vi "database_connection_write.vi"(5 "ODBC data source name":string="amrc_monitoring", 6 "error in (no error)":errorcluster, 7 "G1?":u32, 8 "current time":timestamp, 9 "data 2":dbl[](array[numeric]), 10 "Machine Data":T1={"Zload"="", "Yload"="", "Xload"="", "path_position"="", "Fovr"="", "SspeedOvr"="", "Program Name"="", "Program status"="", "Block of code being executed"="", "Line of code"="", "Machine availability"="", "Emergency status"="", "Controller mode"="", "Tool_id"="UNAVAILABLE"}, 11 "Machine type":string) -> (3 "error out":errorcluster)   [LabVIEW 2017]
uses:
  <vilib>/addons/database/Connection.llb/DB Tools Open Connec (String).vi
  <vilib>/addons/database/Connection.llb/Conn Execute.vi
  <vilib>/addons/database/Recordset.llb/Rec Destroy - Connection.vi
  <vilib>/addons/database/NI_Database_API.lvlib
panel:
  out "Tool_id":string
  out "resulting string":string
  out "size(s)":i32
  out "concatenated string 5":string
  out "concatenated string 4":string
  out "concatenated string 3":string
  out "concatenated string 2":string
  out "concatenated string":string
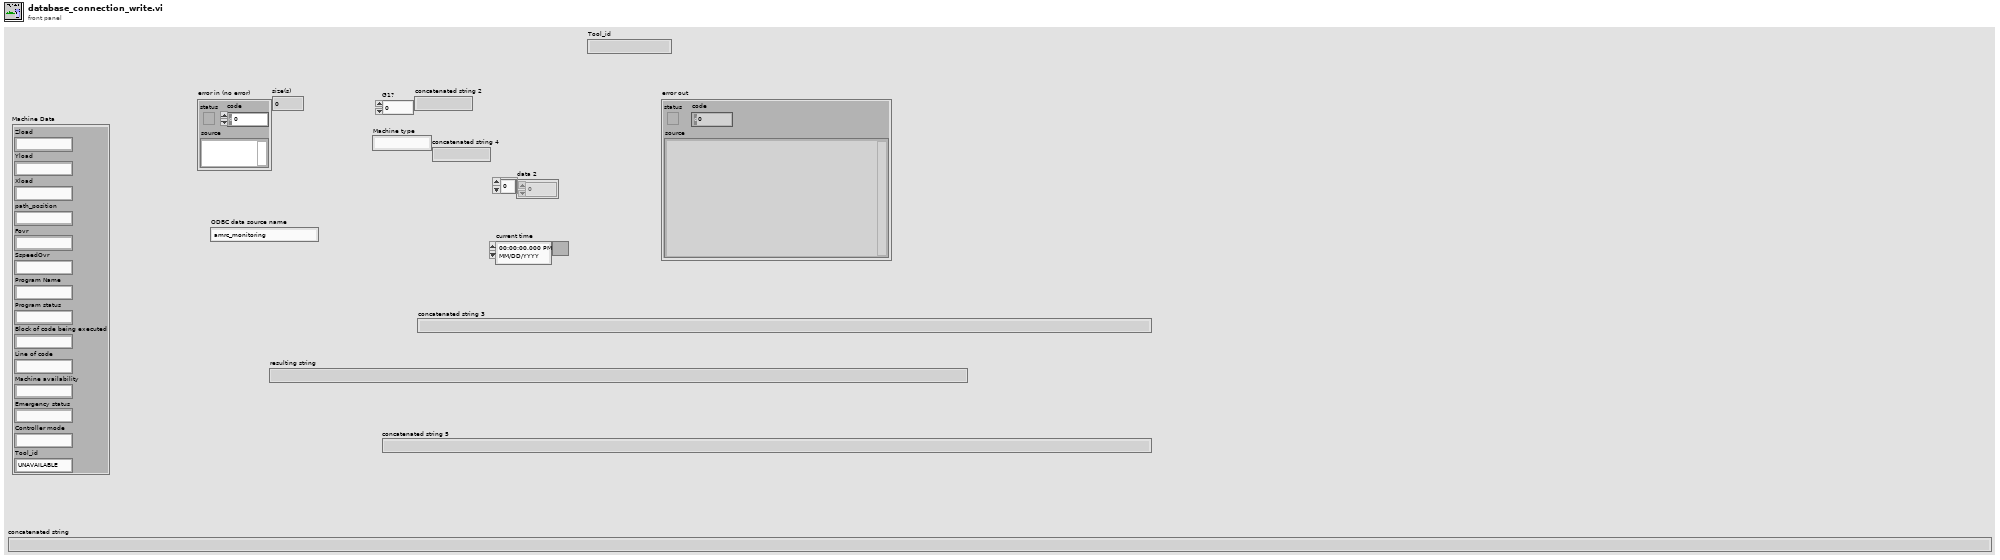
[diagram p1: front panel]
types:
  T1 = cluster{"Zload":string, "Yload":string, "Xload":string, "path_position":string, "Fovr":string, "SspeedOvr":string, "Program Name":string, "Program status":string, "Block of code being executed":string, "Line of code":string, "Machine availability":string, "Emergency status":string, "Controller mode":string, "Tool_id":string}
  T2 = typedef "NI_Database_API.lvlib/Conn ObjectReference.ctl" = refnum<k1>
  T3 = typedef "NI_Database_API.lvlib/Rec ObjectReference.ctl" = refnum<k1>
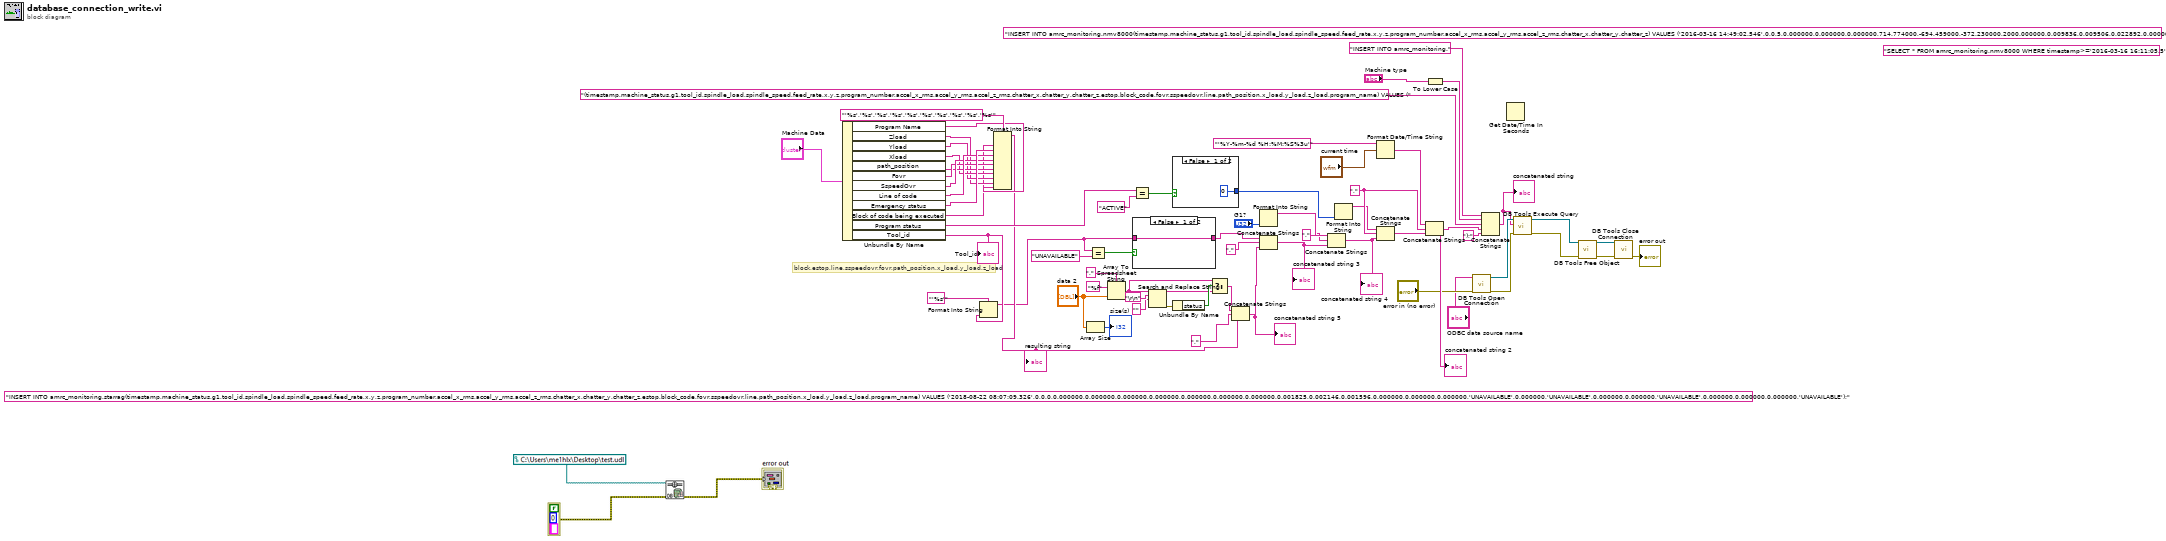
[diagram p0: block diagram]
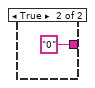
[diagram p2: hidden frame]
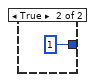
[diagram p3: hidden frame]
diagram:
  (unwired) "INSERT INTO amrc_monitoring.starrag(timestamp,machine_status,g1,tool_id,spindle_load,spindle_speed,feed_rate,x,y,z,program_number,accel_x_rms,accel_y_rms,accel_z_rms,chatter_x,chatter_y,chatter_z,estop,block_code,fovr,sspeedovr,line,path_position,x_load,y_load,z_load,program_name) VALUES ('2018-08-22 08:07:09.326',0,0,0,0.000000,0.000000,0.000000,0.000000,0.000000,0.000000,0.000000,0.001825,0.002146,0.001596,0.000000,0.000000,0.000000,'UNAVAILABLE',0.000000,'UNAVAILABLE',0.000000,0.000000,'UNAVAILABLE',0.000000,0.000000,0.000000,'UNAVAILABLE');" ("string")
  w47 = "," ("string")
  (unwired) "SELECT * FROM amrc_monitoring.nmv8000 WHERE timestamp>='2016-03-16 16:11:05.5' " ("SQL query")
  (unwired) "INSERT INTO amrc_monitoring.nmv8000(timestamp,machine_status,g1,tool_id,spindle_load,spindle_speed,feed_rate,x,y,z,program_number,accel_x_rms,accel_y_rms,accel_z_rms,chatter_x,chatter_y,chatter_z) VALUES ('2016-03-16 14:49:02.546',0,0,5,0.000000,0.000000,0.000000,714.774000,-694.459000,-372.230000,2000.000000,0.009836,0.009506,0.022892,0.000000,1.000000,0.000000);" ("SQL query")
  # "block,estop,line,sspeedovr,fovr,path_position,x_load,y_load,z_load"
  n1 = Unbundle By Name("Machine Data") -> ("Program Name"=w16:string, "Zload"=w21:string, "Yload"=w22:string, "Xload"=w23:string, "path_position"=w24:string, "Fovr"=w25:string, "SspeedOvr"=w26:string, "Line of code"=w27:string, "Emergency status"=w28:string, "Block of code being executed"=w12:string, "Program status"=w57:string, "Tool_id"=w2:string)
  "Tool_id" <- w2
  n2 = Format Into String(format string="'%s'", w2) -> (resulting string=w1:string)  [unwired: 2 in, 1 out]
  n3 = Format Into String(format string="'%s','%s','%s','%s','%s','%s','%s','%s','%s','%s'", w12, w28, w27, w26, w25, w24, w23, w22, w21, w16) -> (resulting string=w6:string)  [unwired: 2 in, 1 out]
  "resulting string" <- w6
  n4 = Array Size(array="data 2") -> (size(s)=→"size(s)":i32)
  n5 = Equal?(x=w1, y="UNAVAILABLE") -> (x = y?=w53:bool)
  n6 = Array To Spreadsheet String(delimiter (Tab)=",", array="data 2", 3:"%f" ("format string")) -> (spreadsheet string=w38:string)
  n7 = case shown="False" w53 {
    tunnel: w1 -> [w65 _]
    tunnel: [w65 "0"] -> w4
    frame False {
    }
    frame True {
    }
  }
  n8 = Equal?(x=w57, y="ACTIVE") -> (x = y?=w55:bool)
  n9 = Search and Replace String(input string=w38, search string="\r\n", replace string="" ("replace string (\"\")")) -> (result string=w39:string, error out=w41:errorcluster)  [unwired: 5 in, 2 out]
  n10 = case shown="False" w55 {
    tunnel: [0 1] -> w54
    frame False {
    }
    frame True {
    }
  }
  n11 = Unbundle By Name(w41) -> ("status"=w40:bool)
  n12 = Select(t=w38, s=w40, f=w39) -> (s? t:f=w18:string)
  n13 = Concatenate Strings(w18, "," ("string"), w6) -> (w17:string)
  "concatenated string 5" <- w17
  n14 = Format Into String("G1?") -> (resulting string=w50:string)  [unwired: 3 in, 1 out]
  n15 = Concatenate Strings(w4, "," ("string"), w17) -> (w10:string)
  "concatenated string 3" <- w10
  n16 = Concatenate Strings(w50, "," ("string"), w10) -> (w15:string)
  "concatenated string 4" <- w15
  n17 = Format Into String(w54) -> (resulting string=w45:string)  [unwired: 3 in, 1 out]
  n18 = Concatenate Strings(w45, w47, w15) -> (w48:string)
  n19 = Format Date/Time String(time format string (%c)="'%Y-%m-%d %H:%M:%S%3u'", seconds (now)="current time") -> (date/time string=w46:string)  [unwired: 1 in]
  n20 = Concatenate Strings(w46, w47, w48) -> (w44:string)
  "concatenated string 2" <- w44
  n21 = To Lower Case(string="Machine type") -> (all lower case string=w35:string)
  n22 = call-poly <vilib>:"DB Tools Open Connection.vi"("error in (no error)"="error in (no error)", "connection information"="ODBC data source name") -> ("error out"=w63:errorcluster, "connection reference"=w64:T2)  [unwired: 6 in]
  n23 = Concatenate Strings("INSERT INTO amrc_monitoring." ("string"), w35, "(timestamp,machine_status,g1,tool_id,spindle_load,spindle_speed,feed_rate,x,y,z,program_number,accel_x_rms,accel_y_rms,accel_z_rms,chatter_x,chatter_y,chatter_z,estop,block_code,fovr,sspeedovr,line,path_position,x_load,y_load,z_load,program_name) VALUES (" ("string"), w44, ");" ("string")) -> (w7:string)
  "concatenated string" <- w7
  n24 = Get Date/Time In Seconds() -> ()  [unwired: 1 out]
  n25 = call-poly <vilib>:"DB Tools Execute Query.vi"("error in (no error)"=w63, "SQL query"=w7, "connection reference"=w64) -> ("error out"=w31:errorcluster, "recordset reference"=w30:T3)  [unwired: 5 in]
  n26 = call-poly <vilib>:"DB Tools Free Object.vi"("error in (no error)"=w31, "recordset reference"=w30) -> ("error out"=w62:errorcluster, "connection reference"=w61:T2)  [unwired: 8 in]
  n27 = call <vilib>:"DB Tools Close Connection.vi"("error in (no error)"=w62, "connection reference"=w61) -> ("error out"=→"error out":errorcluster)  [unwired: 5 in]
